vi "Deactivate All.vi"(8 "error in (no error)":errorcluster, 11 "BME_DG_System in":refnum<class "BME_DG_System.lvclass">) -> (0 "error out":errorcluster, 3 "BME_DG_System out":refnum<class "BME_DG_System.lvclass">)   [LabVIEW 2009, in "BME_DG_System.lvclass"]
uses:
  BME_DG_System.lvclass
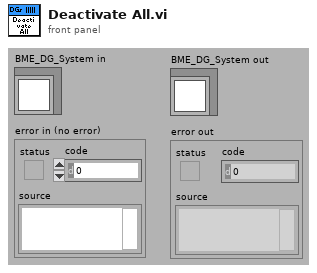
[diagram p1: front panel]
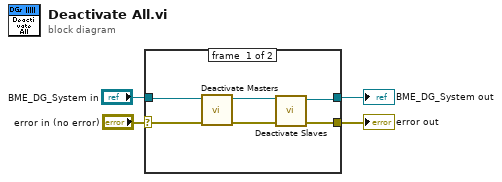
[diagram p0: block diagram]
diagram:
  n1 = case shown="No Error" "error in (no error)" {
    selector: "error in (no error)" -> [w9 w12]
    tunnel: [w5 w12] -> w3
    tunnel: [w6 w11] -> w1
    tunnel: "BME_DG_System in" -> [w10 w11]
    frame #0 {
      n2 = call "Deactivate Masters.vi"("error in (no error)"=w9, "BME_DG_System in"=w10) -> ("error out"=w7:errorcluster, "BME_DG_System out"=w8:refnum<class "BME_DG_System.lvclass">)  [unwired: 8 in]
      n3 = call "Deactivate Slaves.vi"("error in (no error)"=w7, "BME_DG_System in"=w8) -> ("error out"=w5:errorcluster, "BME_DG_System out"=w6:refnum<class "BME_DG_System.lvclass">)  [unwired: 8 in]
    }
    frame #1 {
    }
  }
  "error out" <- w3
  "BME_DG_System out" <- w1
